vi "ACCESS加密 (子VI).vi"(8 "错误输入（无错误）":errorcluster) -> (0 "错误输出":errorcluster)   [LabVIEW 2016]
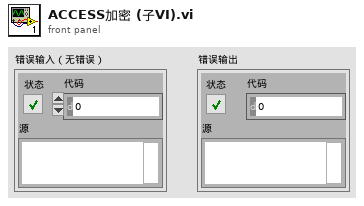
[diagram p1: front panel]
types:
  T1 = typedef "数据库类型.ctl" = enum16{"Access", "SQLite"}
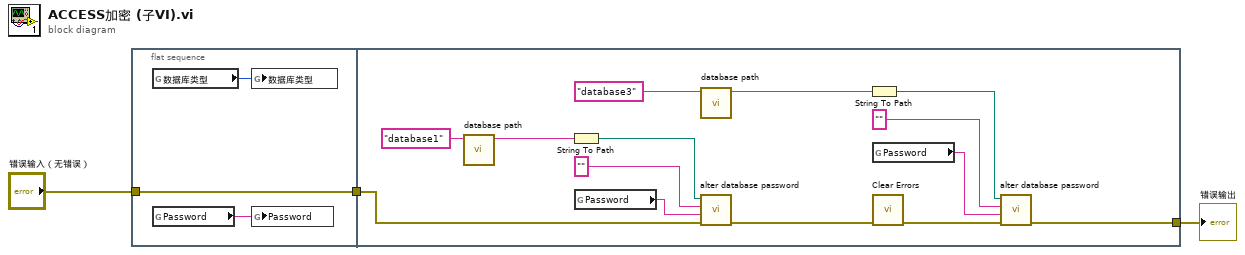
[diagram p0: block diagram]
diagram:
  n1 = flat-sequence {
    tunnel: "错误输入（无错误）" -> [w6]
    tunnel: [w6] -> w1
    tunnel: [w19] -> w2
    tunnel: w1 -> [w20]
    frame #0 {
      n2 = global read "系统设置全局变量.vi" "数据库类型"() -> (w4:T1)
      n3 = global read "系统设置全局变量.vi" "Password"() -> (w5:string)
      n4 = global write "外部调用接口全局变量.vi" "数据库类型"(w4) -> ()
      n5 = global write "外部调用接口全局变量.vi" "Password"(w5) -> ()
    }
    frame #1 {
      n6 = call "database path.vi"("database"="database1") -> ("Path out"=w8:string)  [unwired: 9 in, 1 out]
      n7 = String To Path(string=w8) -> (path=w9:path)
      n8 = global read "系统设置全局变量.vi" "Password"() -> (w11:string)
      n9 = call "database path.vi"("database"="database3") -> ("Path out"=w15:string)  [unwired: 9 in, 1 out]
      n10 = call "alter database password.vi"("错误输入（无错误）"=w20, "NewPWd"=w11, "OpenPwd"="", "路径"=w9) -> ("错误输出"=w17:errorcluster)  [unwired: 7 in]
      n11 = String To Path(string=w15) -> (path=w14:path)
      n12 = global read "系统设置全局变量.vi" "Password"() -> (w12:string)
      n13 = call <vilib>:"Clear Errors.vi"("error in (no error)"=w17) -> ("error out"=w18:errorcluster)  [unwired: 5 in, 1 out]
      n14 = call "alter database password.vi"("错误输入（无错误）"=w18, "NewPWd"=w12, "OpenPwd"="", "路径"=w14) -> ("错误输出"=w19:errorcluster)  [unwired: 7 in]
    }
  }
  "错误输出" <- w2
